vi "cnvrt_THz_waveNr.vi"(0 "frequency (THz)":dbl format="%.2f", 5 "error in (no error)":errorcluster) -> (14 "waveNr/cm":dbl format="%.2f", 19 "error out":errorcluster)   [LabVIEW 2010, in "OSA.lvclass"]
uses:
  OSA.lvclass
  FTSLib.dll
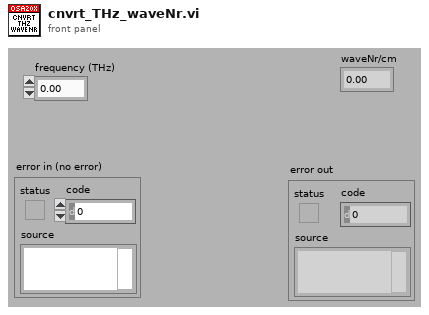
[diagram p1: front panel]
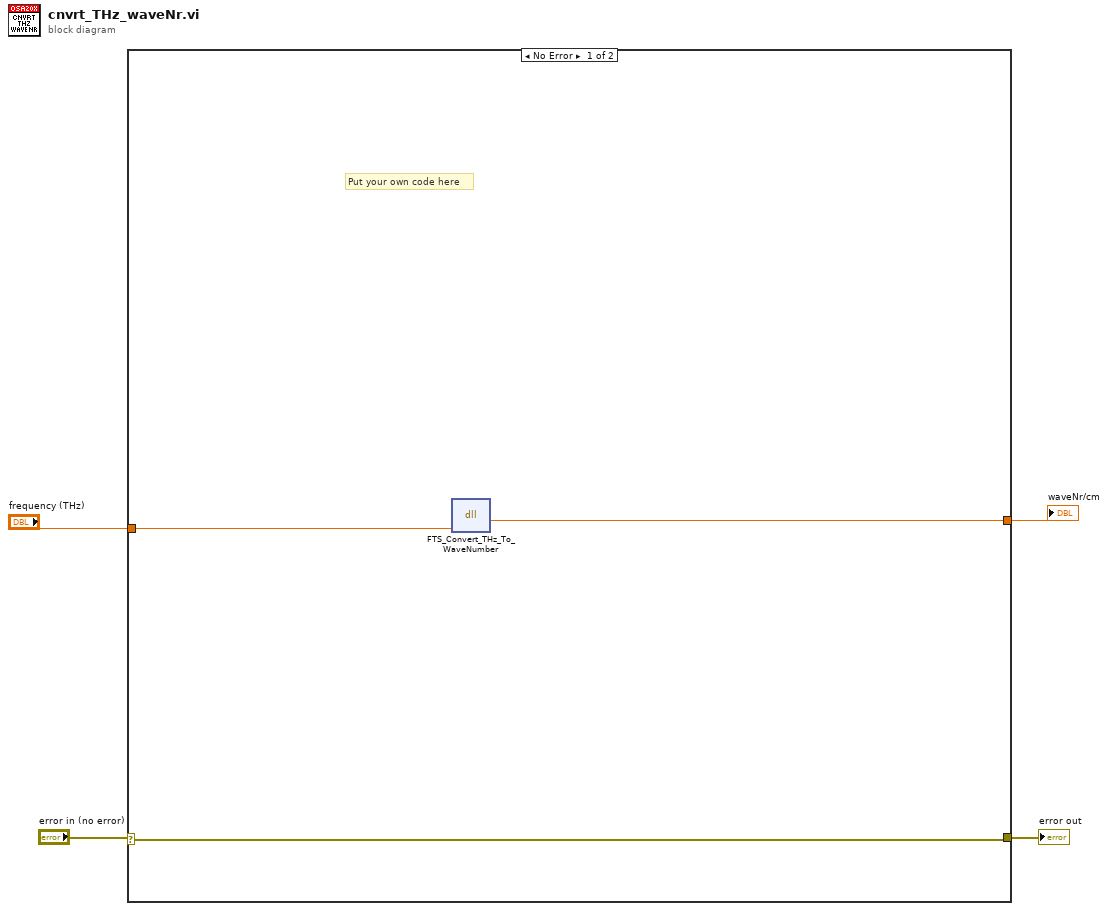
[diagram p0: block diagram]
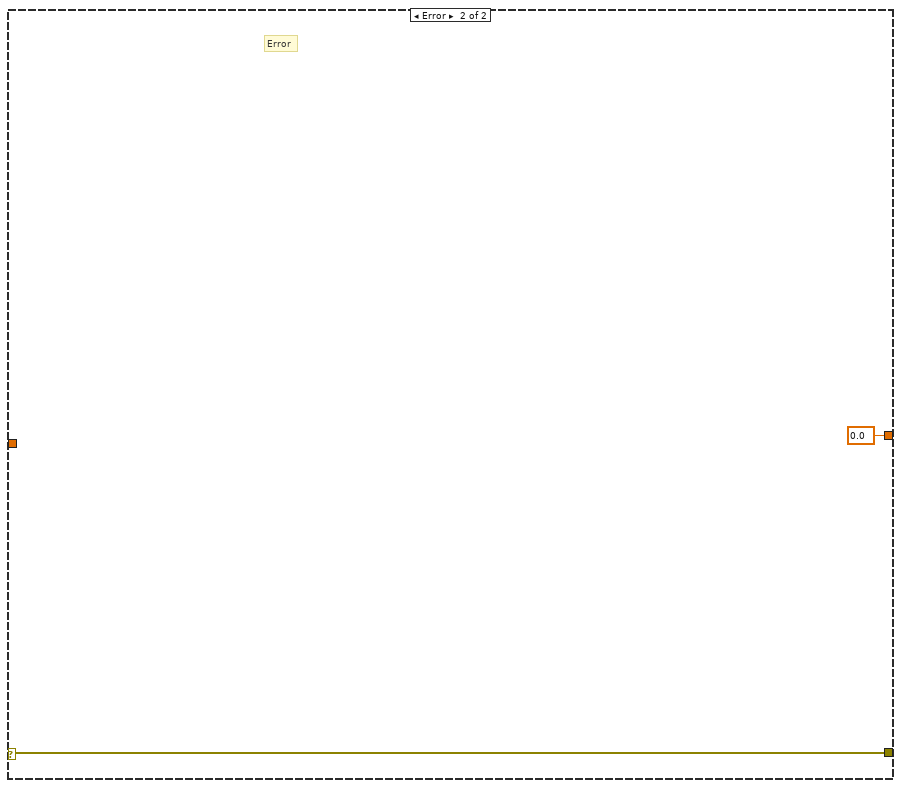
[diagram p2: hidden frame]
diagram:
  n1 = case shown="No Error" "error in (no error)" {
    selector: "error in (no error)" -> [w5 w9]
    tunnel: [w5 w9] -> w4
    tunnel: "frequency (THz)" -> [w7 _]
    tunnel: [w6 0.0] -> w1
    frame No Error {
      # "Put your own code here"
      n2 = dll-call lib="FTSLib.dll" fn="FTS_Convert_THz_To_WaveNumber"("frequency"=w7) -> ("return type"=w6:dbl)  [unwired: 4 in, 2 out]
    }
    frame Error {
      # "Error"
    }
  }
  "error out" <- w4
  "waveNr/cm" <- w1
